vi "Begin.vi"(11 "Image Size":T1=enum."160x120") -> (0 "error out":errorcluster)   [LabVIEW 2012]
doc: "Called before other user functions, this VI is expected to open initial I/O refnums, load in file data, and do all program initialization. Notice that the <B>error out</B> terminal is simply used for data flow. Wiring it to other structures or subVIs ensures that this VI runs first."
uses:
  <vilib>/Rock Robotics/WPI/Camera/WPI_CameraImageSize.ctl
  <vilib>/Rock Robotics/WPI/DriverStation/WPI_DriverStationRobotMode2.ctl
  <vilib>/Rock Robotics/WPI/Joystick/WPI_JoystickDeviceEnum.ctl
  <vilib>/Rock Robotics/SystemInterfaces/AI/FPGA_AIChannel.ctl
  <vilib>/Rock Robotics/SystemInterfaces/Typedef/FPGA_TypedefSolenoidModule.ctl
  <vilib>/Rock Robotics/WPI/Solenoid/WPI_SolenoidChannel.ctl
  <vilib>/Rock Robotics/SystemInterfaces/DIO/FPGA_DIOChannel.ctl
  <vilib>/Rock Robotics/SystemInterfaces/DIO/FPGA_DIOPWMChannel.ctl
  <vilib>/Rock Robotics/WPI/SafetyOutput/WPI_SafetyOutputConfigMenu.ctl
  <vilib>/Rock Robotics/WPI/CAN/Jaguar/SubVIs/WPI_CANJaguar_ControlMode.ctl
  <vilib>/Rock Robotics/SystemInterfaces/Typedef/FPGA_TypedefDigitalModule.ctl
  <vilib>/Rock Robotics/WPI/Solenoid/WPI_SolenoidValue.ctl
  <vilib>/Rock Robotics/SystemInterfaces/DIO/FPGA_DIORelayChannel.ctl
  Robot Global Data.vi
  <vilib>/Rock Robotics/WPI/Solenoid/WPI_SolenoidOpenDouble.vi
  <vilib>/Rock Robotics/WPI/Solenoid/WPI_SolenoidSetEnum.vi
  <vilib>/Rock Robotics/WPI/RobotDrive/WPI_RobotDriveOpen4MotorWithVictor.vi
  <vilib>/Rock Robotics/WPI/MotorControl/WPI_MotorControlOpenCANJaguar.vi
  <vilib>/Rock Robotics/WPI/MotorControl/WPI_MotorControlOpen Victor.vi
  <vilib>/Rock Robotics/WPI/Compressor/WPI_CompressorGetSetRefNum.vi
  <vilib>/Rock Robotics/WPI/Camera/WPI_CameraWhite Balance Values.ctl
  <vilib>/Rock Robotics/WPI/Camera/WPI_CameraExposure Values.ctl
  <vilib>/Rock Robotics/WPI/Camera/WPI_CameraFrameRate.ctl
  <vilib>/Rock Robotics/WPI/Counter/WPI_CounterDigitalInputToDigitalSource.vi
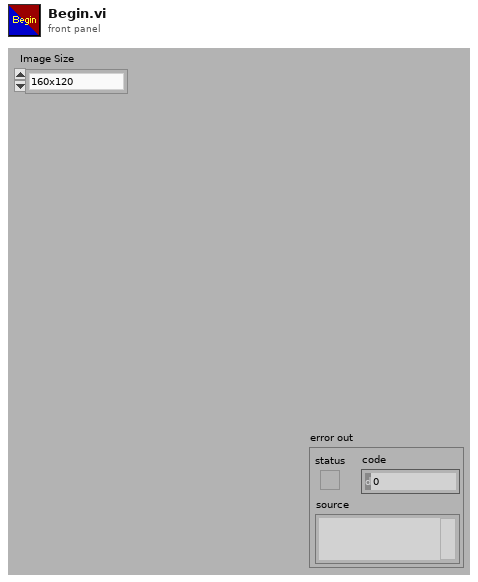
[diagram p1: front panel]
types:
  T1 = typedef "WPI_CameraImageSize.ctl" = enum16{"640x480", "320x240", "160x120"}
  T2 = typedef "FPGA_AIChannel.ctl" = enum8{"AI 1", "AI 2", "AI 3", "AI 4", "AI 5", "AI 6", "AI 7", "AI 8", "Invalid"}
  T3 = typedef "FPGA_DIORelayChannel.ctl" = enum8{"Relay 1", "Relay 2", "Relay 3", "Relay 4", "Relay 5", "Relay 6", "Relay 7", "Relay 8", "Invalid"}
  T4 = typedef "FPGA_TypedefDigitalModule.ctl" = enum16{"Digital Module 1", "Digital Module 2"}
  T5 = typedef "FPGA_DIOChannel.ctl" = enum8{"DIO 1", "DIO 2", "DIO 3", "DIO 4", "DIO 5", "DIO 6", "DIO 7", "DIO 8", "DIO 9", "DIO 10", "DIO 11", "DIO 12", "DIO 13", "DIO 14", "Invalid"}
  T6 = typedef "FPGA_DIOPWMChannel.ctl" = enum8{"PWM 1", "PWM 2", "PWM 3", "PWM 4", "PWM 5", "PWM 6", "PWM 7", "PWM 8", "PWM 9", "PWM 10", "Invalid"}
  T7 = typedef "WPI_SolenoidValue.ctl" = enum16{"Off", "On", "Forward", "Reverse"}
  T8 = typedef "WPI_SolenoidChannel.ctl" = enum8{"Solenoid 1", "Solenoid 2", "Solenoid 3", "Solenoid 4", "Solenoid 5", "Solenoid 6", "Solenoid 7", "Solenoid 8", "Invalid"}
  T9 = typedef "FPGA_TypedefSolenoidModule.ctl" = enum16{"Solenoid Module 1", "Solenoid Module 2"}
  T10 = typedef "WPI_CANJaguar_ControlMode.ctl" = enum8{"Percent VBus", "Current", "Speed", "Position", "Voltage"}
  T11 = typedef "WPI_SafetyOutputConfigMenu.ctl" = enum16{"Enable", "Disable"}
  T12 = typedef "WPI_JoystickDeviceEnum.ctl" = enum16{"USB 1", "USB 2", "USB 3", "USB 4", "Kinect 1", "Kinect 2"}
  T13 = typedef "WPI_DriverStationRobotMode2.ctl" = enum16{"Autonomous Disabled", "Autonomous Enabled", "Teleop Disabled", "Teleop Enabled", "Timeout", "Finish", "Test Disabled", "Test Enabled"}
  T14 = typedef "WPI_CameraFrameRate.ctl" = u32
  T15 = typedef "WPI_CameraExposure Values.ctl" = enum16{"Auto", "Flicker-free 50 Hz", "Flicker-free 60 Hz", "Hold current"}
  T16 = typedef "WPI_CameraWhite Balance Values.ctl" = enum16{"Auto", "Fixed indoor", "Fixed outdoor 1", "Fixed outdoor 2", "Fixed fluorescent 1", "Fixed fluorescent 2", "Hold current"}
  T17 = typedef "WPI_CameraDevRef.ctl" = cluster{"Camera Address":string, "CameraStatus":errorcluster, "Acquire Image Notifier":refnum<notifier>}
  T18 = typedef "WPI_CompressorDevRef.ctl" = cluster{"DevStatus":errorcluster, "DigitalInputDevRef":T19, "RelayDevRef":T20}
  T19 = typedef "WPI_DigitalInputDevRef.ctl" = cluster{"DevStatus":errorcluster, "DIO Channel":T5, "Digital Module":T4}
  T20 = typedef "WPI_RelayDevRef.ctl" = cluster{"DevStatus":errorcluster, "Relay Channel":T3, "Digital Module":T4, "Relay Direction":T21}
  T21 = typedef "WPI_RelayDirection.ctl" = enum16{"Both directions", "Forward only", "Reverse only"}
  T22 = typedef "FPGA_CounterEncoderSourceConvertionLVSourceType.ctl" = cluster{"DevStatus":errorcluster, "AnalogTriggerMode?":bool, "DigitalMode":cluster{"Digital Module":T4, "DIO Channel":T23}, "AnalogTriggerMode":cluster{"AnalogTriggerIndex":T24, "OutputType":T25}}
  T23 = typedef "FPGA_DIODigitalSourceChannel.ctl" = enum8{"DIO 1", "DIO 2", "DIO 3", "DIO 4", "DIO 5", "DIO 6", "DIO 7", "DIO 8", "DIO 9", "DIO 10", "DIO 11", "DIO 12", "DIO 13", "DIO 14", "Disabled"}
  T24 = typedef "FPGA_AnalogTriggerIndex.ctl" = enum8{"Trig 0", "Trig 1", "Trig 2", "Trig 3", "Trig 4", "Trig 5", "Trig 6", "Trig 7", "Invalid"}
  T25 = typedef "FPGA_AnalogTriggerOutType.ctl" = enum16{"InWindow", "TriggerState", "Rising", "Falling"}
  T26 = typedef "WPI_EncoderDevRef.ctl" = cluster{"DevStatus":errorcluster, "EncoderIndex":T27, "CounterIndex":T28, "DistancePerCount":dbl, "Decoding Type":T29}
  T27 = typedef "FPGA_EncoderIdx.ctl" = enum8{"Enc 0", "Enc 1", "Enc 2", "Enc 3", "Invalid"}
  T28 = typedef "FPGA_CounterCtrSystemIndex.ctl" = enum8{"Ctr 0", "Ctr 1", "Ctr 2", "Ctr 3", "Ctr 4", "Ctr 5", "Ctr 6", "Ctr 7", "Invalid"}
  T29 = typedef "WPI_EncoderType.ctl" = enum16{"1x", "2x", "4x"}
  T30 = typedef "WPI_JoystickDevRef.ctl" = cluster{"Device":T12}
  T31 = typedef "WPI_AnalogChannelDevRef.ctl" = cluster{"DevStatus":errorcluster, "Analog Module":T32, "Analog Channel":T2}
  T32 = typedef "FPGA_TypedefAnalogModule.ctl" = enum16{"Analog Module 1", "Analog Module 2"}
  T33 = typedef "WPI_MotorControlDeviceRef.ctl" = cluster{"DeviceStatus":errorcluster, "Type":enum16{"PWM", "CAN"}, "PWM":cluster{"Digital Module":T4, "PWM Channel":T6, "DeadBand":T34}, "CAN":cluster{"Device Number":u8, "Control Mode":T10, "Semaphore":T35, "Max Vout":dbl}, "Invert":bool, "TransformRef":T36, "InvTransformRef":T36}
  T34 = typedef "WPI_PWMDeadband.ctl" = cluster{"Name":string, "maxPositivePwm":i32, "minPositivePwm":i32, "centerPwm":i32, "maxNegativePwm":i32, "minNegativePwm":i32, "angularRange":u16}
  T35 = typedef "Semaphore RefNum" = refnum<k1>
  T36 = typedef "WPI_PWMTransform_ConPane.ctl" = refnum<vi>
  T37 = typedef "WPI_SolenoidDevRef.ctl" = cluster{"DevStatus":errorcluster, "Solenoid Module":T9, "Forward Solenoid Channel":T8, "Reverse Solenoid Channel":T8}
  T38 = typedef "WPI_RobotDriveDevRef.ctl" = cluster{"DevStatus":errorcluster, "Motors[]":T33[], "Square Inputs":bool, "Max Output":dbl, "Isochronous":bool}
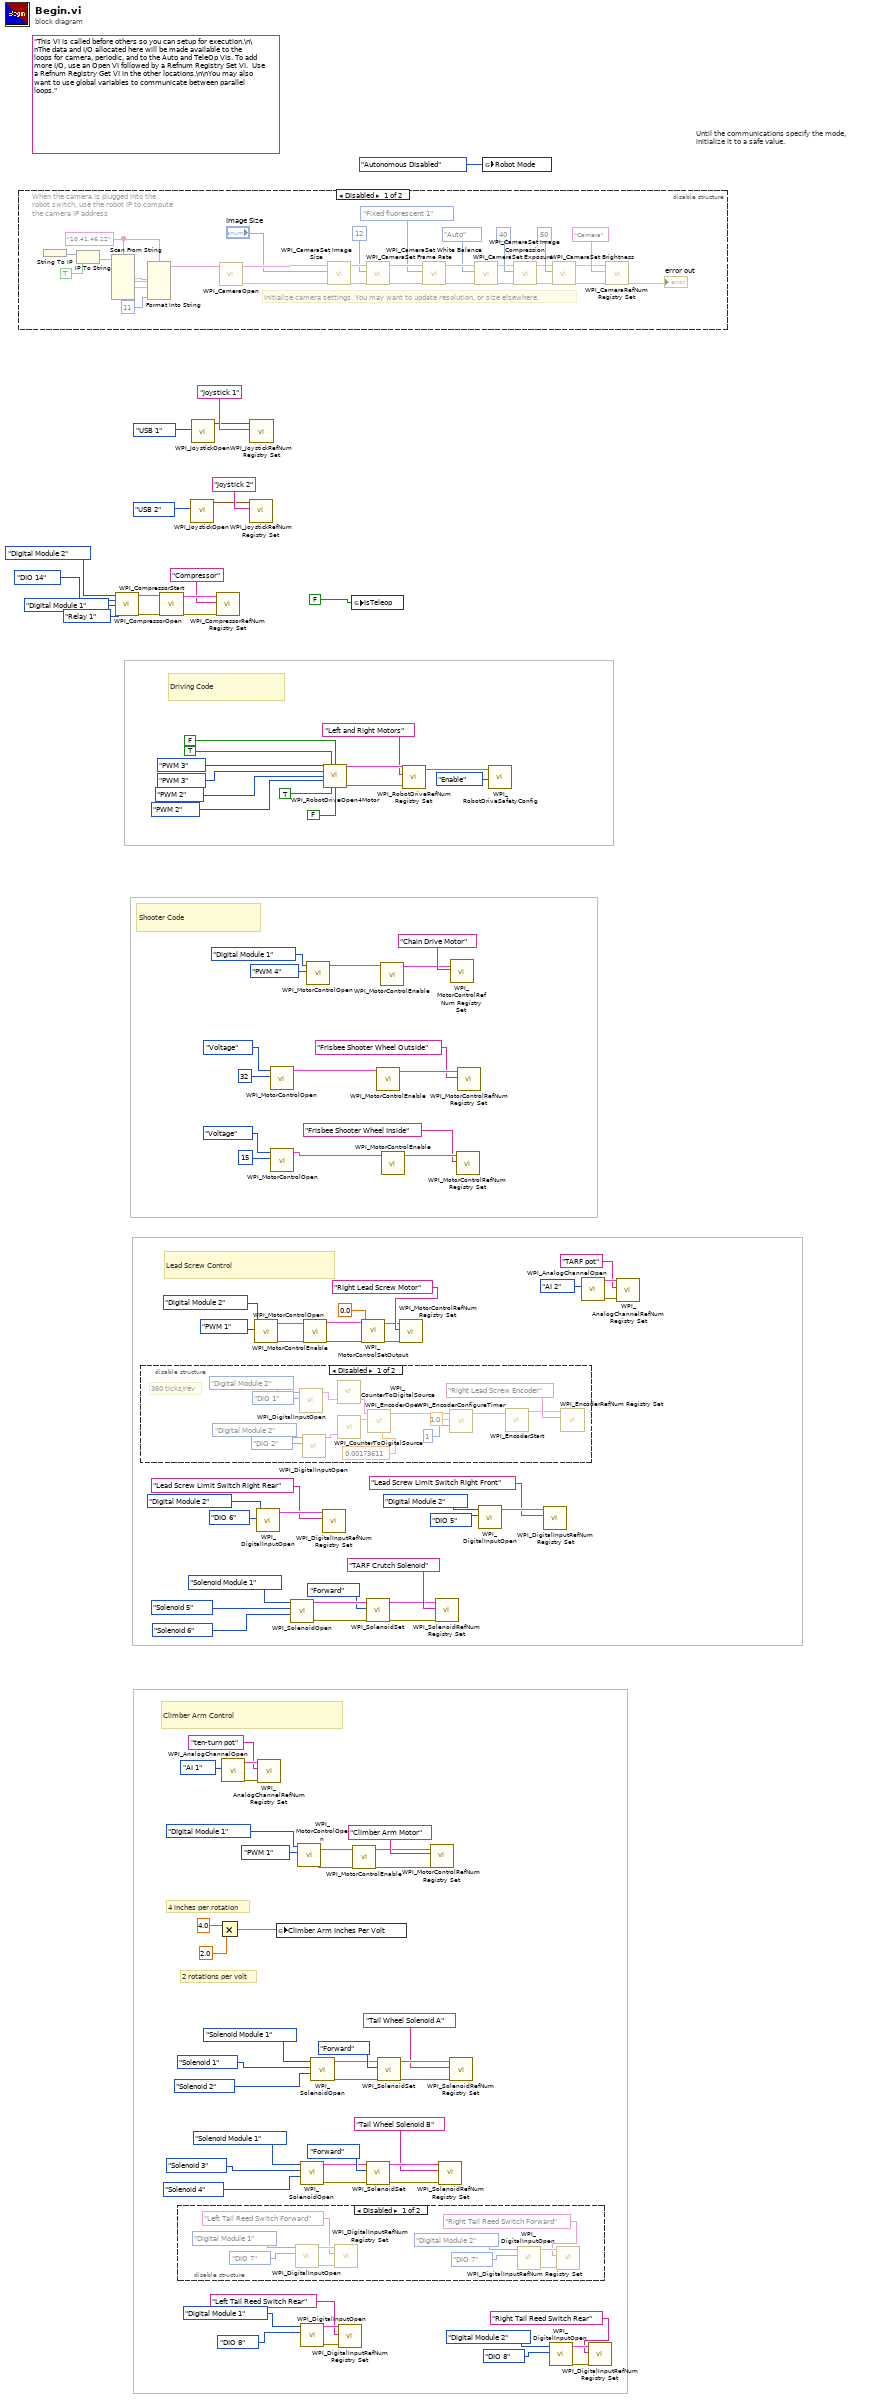
[diagram p0: block diagram]
diagram:
  (unwired) "This VI is called before others so you can setup for execution.\n\nThe data and I/O allocated here will be made available to the loops for camera, periodic, and to the Auto and TeleOp VIs. To add more I/O, use an Open VI followed by a Refnum Registry Set VI.  Use a Refnum Registry Get VI in the other locations.\n\nYou may also want to use global variables to communicate between parallel loops."
  # "Lead Screw Control"
  # "Shooter Code"
  # "Driving Code"
  # "2 rotations per volt"
  # "4 inches per rotation"
  # "Climber Arm Control"
  # "Until the communications specify the mode,\ninitialize it to a safe value."
  n1 = disable-structure shown="Disabled" {
    frame Disabled {
      w121 = "10.41.46.12" ("format string")
      # "When the camera is plugged into the\nrobot switch, use the robot IP to compute\nthe camera IP address"
      # "Initialize camera settings. You may want to update resolution, or size elsewhere."
      n2 = String To IP() -> (0:w128:u32)  [unwired: 1 in]
      n3 = IP To String(1:TRUE ("dot notation? (F)"), 2:w128) -> (0:w126:string)
      n4 = Scan From String(format string=w121, input string=w126) -> (output 1=w125, output 2=w124, output 3=w123)  [unwired: 7 in, 3 out]
      n5 = Format Into String(format string=w121, w125, w124, w123, 11 ("Compression")) -> (resulting string=w120:string)  [unwired: 2 in, 1 out]
      n6 = call <vilib>:"WPI_CameraOpen.vi"("Camera Address"=w120) -> ("error out"=w140:errorcluster, "CameraDevRef"=w141:T17)  [unwired: 1 in, 8 out]
      n7 = call <vilib>:"WPI_CameraSet Image Size.vi"("error in (no error)"=w140, "Image Size"="Image Size", "CameraDevRef"=w141) -> ("error out"=w139:errorcluster, "CameraDevRef Out"=w142:T17)  [unwired: 7 out]
      n8 = call <vilib>:"WPI_CameraSet Frame Rate.vi"("error in (no error)"=w139, "Frame Rate (fps)"=T14 12, "CameraDevRef"=w142) -> ("error out"=w138:errorcluster, "CameraDevRef Out"=w144:T17)  [unwired: 7 out]
      n9 = call <vilib>:"WPI_CameraSet White Balance.vi"("error in (no error)"=w138, "White Balance"=WPI_CameraWhite_Balance_Values."Fixed fluorescent 1", "CameraDevRef"=w144) -> ("error out"=w137:errorcluster, "CameraDevRef Out"=w143:T17)  [unwired: 7 out]
      n10 = call <vilib>:"WPI_CameraSet Exposure.vi"("error in (no error)"=w137, "Exposure"=WPI_CameraExposure_Values."Auto", "CameraDevRef"=w143) -> ("error out"=w136:errorcluster, "CameraDevRef Out"=w146:T17)  [unwired: 7 out]
      n11 = call <vilib>:"WPI_CameraSet Image Compression.vi"("error in (no error)"=w136, "Compression"=40, "CameraDevRef"=w146) -> ("error out"=w135:errorcluster, "CameraDevRef Out"=w145:T17)  [unwired: 7 out]
      n12 = call <vilib>:"WPI_CameraSet Brightness.vi"("error in (no error)"=w135, "Brightness"=50, "CameraDevRef"=w145) -> ("error out"=w133:errorcluster, "CameraDevRef Out"=w134:T17)  [unwired: 7 out]
      n13 = call <vilib>:"WPI_CameraRefNum Registry Set.vi"("error in (no error)"=w133, "refnum name"="Camera", "CameraDevRef"=w134) -> ("error out"=→"error out":errorcluster)  [unwired: 8 out]
    }
    frame Enabled {
    }
  }
  n14 = call <vilib>:"WPI_CompressorOpen.vi"("Pressure Switch Digital Module (Module 1)"=FPGA_TypedefDigitalModule."Digital Module 2", "Pressure Switch DIO Channel"=FPGA_DIOChannel."DIO 14", "Relay Digital Module (Module 1)"=FPGA_TypedefDigitalModule."Digital Module 1", "Relay Channel"=FPGA_DIORelayChannel."Relay 1") -> ("CompressorDevRef"=w18:T18, "error out"=w19:errorcluster)  [unwired: 10 in]
  n15 = disable-structure shown="Disabled" {
    frame Disabled {
      # "360 ticks/rev"
      n16 = call <vilib>:"WPI_DigitalInputOpen.vi"("DIO Channel"=FPGA_DIOChannel."DIO 1", "Digital Module (Module 1)"=FPGA_TypedefDigitalModule."Digital Module 2") -> ("DigitalInputDevRef"=w151:T19)  [unwired: 8 in, 1 out]
      n17 = call <vilib>:"WPI_DigitalInputOpen.vi"("DIO Channel"=FPGA_DIOChannel."DIO 2", "Digital Module (Module 1)"=FPGA_TypedefDigitalModule."Digital Module 2") -> ("DigitalInputDevRef"=w150:T19)  [unwired: 8 in, 1 out]
      n18 = call-poly <vilib>:"WPI_CounterToDigitalSource.vi"("DigitalInputDevRef"=w151) -> ("Digital Source"=w159:T22)  [unwired: 6 in]
      n19 = call-poly <vilib>:"WPI_CounterToDigitalSource.vi"("DigitalInputDevRef"=w150) -> ("Digital Source"=w160:T22)  [unwired: 6 in]
      n20 = call <vilib>:"WPI_EncoderOpen.vi"("DistancePerCount"=0.00173611 ("Distance Per Line(in.)"), "BSource"=w160, "ASource"=w159) -> ("EncoderDevRef"=w161:T26)  [unwired: 7 in, 1 out]
      n21 = call <vilib>:"WPI_EncoderConfigureTimer.vi"("Number Samples to Average"=u8 1, "Minimum Rate"=1.0, "EncoderDevRef"=w161) -> ("EncoderDevRef"=w162:T26)  [unwired: 7 in, 1 out]
      n22 = call <vilib>:"WPI_EncoderStart.vi"("EncoderDevRef"=w162) -> ("EncoderDevRef"=w163:T26)  [unwired: 9 in, 1 out]
      n23 = call <vilib>:"WPI_EncoderRefNum Registry Set.vi"("refnum name"="Right Lead Screw Encoder", "EncoderDevRef"=w163) -> ()  [unwired: 8 in, 2 out]
    }
    frame Enabled {
    }
  }
  n24 = call <vilib>:"WPI_CompressorStart.vi"("error in (no error)"=w19, "CompressorDevRef"=w18) -> ("error out"=w17:errorcluster, "CompressorDevRef"=w16:T18)  [unwired: 8 in]
  n25 = disable-structure shown="Disabled" {
    frame Disabled {
      n26 = call <vilib>:"WPI_DigitalInputOpen.vi"("DIO Channel"=FPGA_DIOChannel."DIO 7", "Digital Module (Module 1)"=FPGA_TypedefDigitalModule."Digital Module 1") -> ("error out"=w174:errorcluster, "DigitalInputDevRef"=w173:T19)  [unwired: 8 in]
      n27 = call <vilib>:"WPI_DigitalInputRefNum Registry Set.vi"("error in (no error)"=w174, "refnum name"="Left Tail Reed Switch Forward", "DigitalInputDevRef"=w173) -> ()  [unwired: 7 in, 2 out]
      n28 = call <vilib>:"WPI_DigitalInputOpen.vi"("DIO Channel"=FPGA_DIOChannel."DIO 7", "Digital Module (Module 1)"=FPGA_TypedefDigitalModule."Digital Module 2") -> ("error out"=w169:errorcluster, "DigitalInputDevRef"=w168:T19)  [unwired: 8 in]
      n29 = call <vilib>:"WPI_DigitalInputRefNum Registry Set.vi"("error in (no error)"=w169, "refnum name"="Right Tail Reed Switch Forward", "DigitalInputDevRef"=w168) -> ()  [unwired: 7 in, 2 out]
    }
    frame Enabled {
    }
  }
  n30 = call <vilib>:"WPI_JoystickOpen.vi"("JoystickDevice"=WPI_JoystickDeviceEnum."USB 2") -> ("JoystickDevRef"=w113:T30)  [unwired: 10 in]
  n31 = call <vilib>:"WPI_JoystickOpen.vi"("JoystickDevice"=WPI_JoystickDeviceEnum."USB 1") -> ("JoystickDevRef"=w116:T30)  [unwired: 10 in]
  n32 = call <vilib>:"WPI_CompressorRefNum Registry Set.vi"("error in (no error)"=w17, "refnum name"="Compressor", "CompressorDevRef"=w16) -> ()  [unwired: 7 in, 2 out]
  n33 = Multiply(x=4.0, y=2.0) -> (x*y=w105:dbl)
  n34 = call <vilib>:"WPI_AnalogChannelOpen.vi"("Analog Channel"=FPGA_AIChannel."AI 1") -> ("error out"=w110:errorcluster, "AIDeviceRef"=w109:T31)  [unwired: 9 in]
  n35 = call <vilib>:"WPI_JoystickRefNum Registry Set.vi"("refnum name"="Joystick 2", "JoystickDevRef"=w113) -> ()  [unwired: 8 in, 2 out]
  n36 = call <vilib>:"WPI_JoystickRefNum Registry Set.vi"("refnum name"="Joystick 1", "JoystickDevRef"=w116) -> ()  [unwired: 8 in, 2 out]
  n37 = call-poly <vilib>:"WPI_MotorControlOpen.vi"("PWM Channel"=FPGA_DIOPWMChannel."PWM 1", "Digital Module (Module 1)"=FPGA_TypedefDigitalModule."Digital Module 2") -> ("error out"=w47:errorcluster, "MotorControlDeviceRef"=w46:T33)  [unwired: 8 in]
  n38 = call <vilib>:"WPI_DigitalInputOpen.vi"("DIO Channel"=FPGA_DIOChannel."DIO 6", "Digital Module (Module 1)"=FPGA_TypedefDigitalModule."Digital Module 2") -> ("DigitalInputDevRef"=w43:T19)  [unwired: 8 in, 1 out]
  n39 = call <vilib>:"WPI_AnalogChannelRefNum Registry Set.vi"("error in (no error)"=w110, "refnum name"="ten-turn pot", "AIDeviceRef"=w109) -> ()  [unwired: 7 in, 2 out]
  n40 = call-poly <vilib>:"WPI_MotorControlOpen.vi"("Device Number"=u8 32, "Control Mode"=WPI_CANJaguar_ControlMode."Voltage") -> ("MotorControlDeviceRef"=w57:T33)  [unwired: 8 in, 1 out]
  n41 = call-poly <vilib>:"WPI_MotorControlOpen.vi"("Device Number"=u8 15, "Control Mode"=WPI_CANJaguar_ControlMode."Voltage") -> ("MotorControlDeviceRef"=w56:T33)  [unwired: 8 in, 1 out]
  n42 = global write "Robot Global Data.vi" "Climber Arm Inches Per Volt"(w105) -> ()
  n43 = call-poly <vilib>:"WPI_SolenoidOpen.vi"("Reverse Solenoid Channel"=WPI_SolenoidChannel."Solenoid 6", "Forward Solenoid Channel"=WPI_SolenoidChannel."Solenoid 5", "Solenoid Module (Module 1)"=FPGA_TypedefSolenoidModule."Solenoid Module 1") -> ("error out"=w31:errorcluster, "SolenoidDevRef"=w30:T37)  [unwired: 7 in]
  n44 = call-poly <vilib>:"WPI_MotorControlOpen.vi"("PWM Channel"=FPGA_DIOPWMChannel."PWM 1", "Digital Module (Module 1)"=FPGA_TypedefDigitalModule."Digital Module 1") -> ("error out"=w22:errorcluster, "MotorControlDeviceRef"=w23:T33)  [unwired: 8 in]
  n45 = call-poly <vilib>:"WPI_SolenoidOpen.vi"("Reverse Solenoid Channel"=WPI_SolenoidChannel."Solenoid 4", "Forward Solenoid Channel"=WPI_SolenoidChannel."Solenoid 3", "Solenoid Module (Module 1)"=FPGA_TypedefSolenoidModule."Solenoid Module 1") -> ("error out"=w91:errorcluster, "SolenoidDevRef"=w90:T37)  [unwired: 7 in]
  n46 = call <vilib>:"WPI_DigitalInputOpen.vi"("DIO Channel"=FPGA_DIOChannel."DIO 8", "Digital Module (Module 1)"=FPGA_TypedefDigitalModule."Digital Module 1") -> ("error out"=w85:errorcluster, "DigitalInputDevRef"=w86:T19)  [unwired: 8 in]
  n47 = call <vilib>:"WPI_MotorControlEnable.vi"("error in (no error)"=w47, "CAN Jaguar Ref"=w46) -> ("error out"=w9:errorcluster, "CAN Jaguar Ref Out"=w10:T33)  [unwired: 8 in]
  n48 = call-poly <vilib>:"WPI_MotorControlOpen.vi"("PWM Channel"=FPGA_DIOPWMChannel."PWM 4", "Digital Module (Module 1)"=FPGA_TypedefDigitalModule."Digital Module 1") -> ("MotorControlDeviceRef"=w61:T33)  [unwired: 8 in, 1 out]
  n49 = call-poly <vilib>:"WPI_SolenoidOpen.vi"("Reverse Solenoid Channel"=WPI_SolenoidChannel."Solenoid 2", "Forward Solenoid Channel"=WPI_SolenoidChannel."Solenoid 1", "Solenoid Module (Module 1)"=FPGA_TypedefSolenoidModule."Solenoid Module 1") -> ("error out"=w100:errorcluster, "SolenoidDevRef"=w99:T37)  [unwired: 7 in]
  n50 = call <vilib>:"WPI_DigitalInputRefNum Registry Set.vi"("refnum name"="Lead Screw Limit Switch Right Rear", "DigitalInputDevRef"=w43) -> ()  [unwired: 8 in, 2 out]
  n51 = call-poly <vilib>:"WPI_RobotDriveOpen4Motor.vi"("Rear Left Motor"=FPGA_DIOPWMChannel."PWM 3" ("Left Motor"), "Rear Left Motor Inverted"=TRUE ("LeftMotorInverted"), "Rear Right Motor Inverted"=FALSE ("RightMotorInverted"), "Rear Right Motor"=FPGA_DIOPWMChannel."PWM 3" ("Right Motor"), "Front Left Motor"=FPGA_DIOPWMChannel."PWM 2", "Front Right Motor"=FPGA_DIOPWMChannel."PWM 2", "Front Left Motor Inverted"=TRUE, "Front Right Motor Inverted"=FALSE) -> ("RobotDriveDevRef"=w74:T38, "error out"=w72:errorcluster)  [unwired: 6 in]
  n52 = call <vilib>:"WPI_DigitalInputRefNum Registry Set.vi"("error in (no error)"=w85, "refnum name"="Left Tail Reed Switch Rear", "DigitalInputDevRef"=w86) -> ()  [unwired: 7 in, 2 out]
  n53 = global write "Robot Global Data.vi" "IsTeleop"(FALSE ("InTeleop")) -> ()
  n54 = call <vilib>:"WPI_MotorControlEnable.vi"("error in (no error)"=w22, "CAN Jaguar Ref"=w23) -> ("error out"=w20:errorcluster, "CAN Jaguar Ref Out"=w21:T33)  [unwired: 8 in]
  n55 = call <vilib>:"WPI_MotorControlSetOutput.vi"("error in (no error)"=w9, "Output"=0.0, "MotorControlDevRef"=w10) -> ("error out"=w6:errorcluster, "MotorControlDevRef"=w7:T33)  [unwired: 6 in, 1 out]
  n56 = call-poly <vilib>:"WPI_SolenoidSet.vi"("error in (no error)"=w31, "Value"=WPI_SolenoidValue."Forward", "SolenoidDevRef"=w30) -> ("error out"=w28:errorcluster, "SolenoidDevRef"=w29:T37)  [unwired: 7 in]
  n57 = call-poly <vilib>:"WPI_SolenoidSet.vi"("error in (no error)"=w91, "Value"=WPI_SolenoidValue."Forward", "SolenoidDevRef"=w90) -> ("error out"=w93:errorcluster, "SolenoidDevRef"=w92:T37)  [unwired: 7 in]
  n58 = call <vilib>:"WPI_MotorControlEnable.vi"("CAN Jaguar Ref"=w57) -> ("CAN Jaguar Ref Out"=w55:T33)  [unwired: 9 in, 1 out]
  n59 = call-poly <vilib>:"WPI_SolenoidSet.vi"("error in (no error)"=w100, "Value"=WPI_SolenoidValue."Forward", "SolenoidDevRef"=w99) -> ("error out"=w102:errorcluster, "SolenoidDevRef"=w101:T37)  [unwired: 7 in]
  n60 = call <vilib>:"WPI_MotorControlEnable.vi"("CAN Jaguar Ref"=w61) -> ("CAN Jaguar Ref Out"=w60:T33)  [unwired: 9 in, 1 out]
  n61 = call <vilib>:"WPI_MotorControlEnable.vi"("CAN Jaguar Ref"=w56) -> ("CAN Jaguar Ref Out"=w54:T33)  [unwired: 9 in, 1 out]
  n62 = call <vilib>:"WPI_MotorControlRefNum Registry Set.vi"("error in (no error)"=w6, "refnum name"="Right Lead Screw Motor", "MotorControlDevRef"=w7) -> ()  [unwired: 7 in, 2 out]
  n63 = call <vilib>:"WPI_RobotDriveRefNum Registry Set.vi"("error in (no error)"=w72, "refnum name"="Left and Right Motors", "RobotDriveDevRef"=w74) -> ("RobotDriveDevRef"=w69:T38)  [unwired: 8 out]
  n64 = call <vilib>:"WPI_MotorControlRefNum Registry Set.vi"("error in (no error)"=w20, "refnum name"="Climber Arm Motor", "MotorControlDevRef"=w21) -> ()  [unwired: 7 in, 2 out]
  n65 = call <vilib>:"WPI_SolenoidRefNum Registry Set.vi"("error in (no error)"=w28, "refnum name"="TARF Crutch Solenoid", "SolenoidDevRef"=w29) -> ()  [unwired: 7 in, 2 out]
  n66 = call <vilib>:"WPI_SolenoidRefNum Registry Set.vi"("error in (no error)"=w93, "refnum name"="Tail Wheel Solenoid B", "SolenoidDevRef"=w92) -> ()  [unwired: 7 in, 2 out]
  n67 = call <vilib>:"WPI_SolenoidRefNum Registry Set.vi"("error in (no error)"=w102, "refnum name"="Tail Wheel Solenoid A", "SolenoidDevRef"=w101) -> ()  [unwired: 7 in, 2 out]
  n68 = call <vilib>:"WPI_MotorControlRefNum Registry Set.vi"("refnum name"="Chain Drive Motor", "MotorControlDevRef"=w60) -> ()  [unwired: 8 in, 2 out]
  n69 = call <vilib>:"WPI_MotorControlRefNum Registry Set.vi"("refnum name"="Frisbee Shooter Wheel Inside", "MotorControlDevRef"=w54) -> ()  [unwired: 8 in, 2 out]
  n70 = call <vilib>:"WPI_MotorControlRefNum Registry Set.vi"("refnum name"="Frisbee Shooter Wheel Outside", "MotorControlDevRef"=w55) -> ()  [unwired: 8 in, 2 out]
  n71 = call <vilib>:"WPI_DigitalInputOpen.vi"("DIO Channel"=FPGA_DIOChannel."DIO 5", "Digital Module (Module 1)"=FPGA_TypedefDigitalModule."Digital Module 2") -> ("DigitalInputDevRef"=w40:T19)  [unwired: 8 in, 1 out]
  n72 = global write "Robot Global Data.vi" "Robot Mode"(WPI_DriverStationRobotMode2."Autonomous Disabled" ("Robot Mode")) -> ()
  n73 = call <vilib>:"WPI_RobotDriveSafetyConfig.vi"("mode"=WPI_SafetyOutputConfigMenu."Enable", "RobotDriveDevRef"=w69) -> ()  [unwired: 8 in, 2 out]
  n74 = call <vilib>:"WPI_DigitalInputRefNum Registry Set.vi"("refnum name"="Lead Screw Limit Switch Right Front", "DigitalInputDevRef"=w40) -> ()  [unwired: 8 in, 2 out]
  n75 = call <vilib>:"WPI_DigitalInputOpen.vi"("DIO Channel"=FPGA_DIOChannel."DIO 8", "Digital Module (Module 1)"=FPGA_TypedefDigitalModule."Digital Module 2") -> ("error out"=w81:errorcluster, "DigitalInputDevRef"=w80:T19)  [unwired: 8 in]
  n76 = call <vilib>:"WPI_AnalogChannelOpen.vi"("Analog Channel"=FPGA_AIChannel."AI 2") -> ("error out"=w4:errorcluster, "AIDeviceRef"=w3:T31)  [unwired: 9 in]
  n77 = call <vilib>:"WPI_DigitalInputRefNum Registry Set.vi"("error in (no error)"=w81, "refnum name"="Right Tail Reed Switch Rear", "DigitalInputDevRef"=w80) -> ()  [unwired: 7 in, 2 out]
  n78 = call <vilib>:"WPI_AnalogChannelRefNum Registry Set.vi"("error in (no error)"=w4, "refnum name"="TARF pot", "AIDeviceRef"=w3) -> ()  [unwired: 7 in, 2 out]
